vi "Read Config.vi"(8 "error in (no error)":errorcluster, 11 "MQTTclient in":refnum<class "MQTTclient.lvclass">) -> (0 "error out":errorcluster, 2 "Config":T1, 3 "MQTTclient out":refnum<class "MQTTclient.lvclass">)   [LabVIEW 2015, in "MQTTclient.lvclass"]
uses:
  MQTTclient.lvclass
  config.ctl
  MQTTclient.lvclass/MQTTclient.ctl
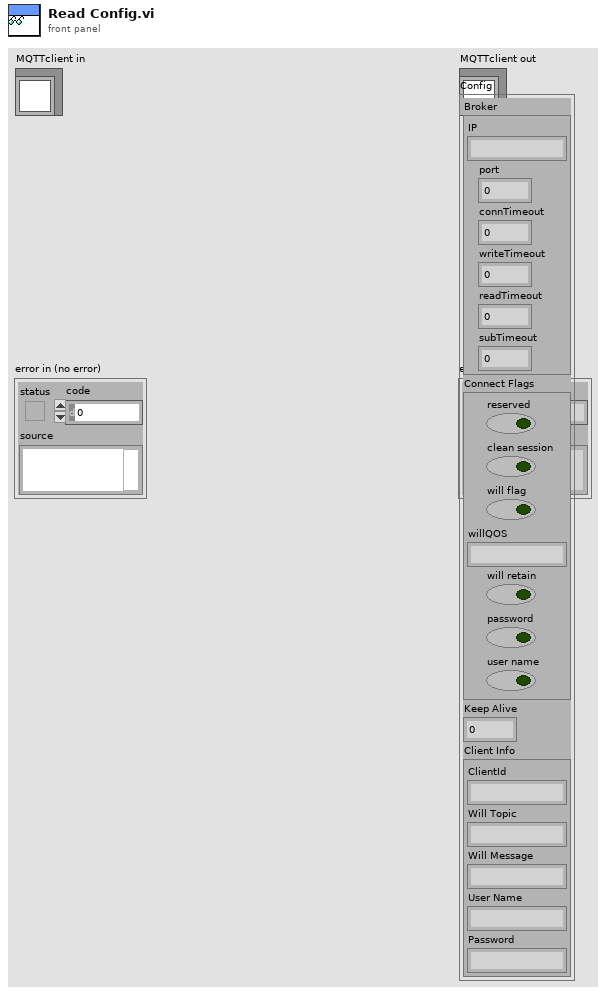
[diagram p1: front panel]
types:
  T1 = typedef "MQTTclient.lvclass/config.ctl" = cluster{"Broker":cluster{"IP":string, "port":u16, "connTimeout":i32, "writeTimeout":i32, "readTimeout":i32, "subTimeout":i32}, "Connect Flags":cluster{"reserved":bool, "clean session":bool, "will flag":bool, "willQOS":string, "will retain":bool, "password":bool, "user name":bool}, "Keep Alive":u16, "Client Info":cluster{"ClientId":string, "Will Topic":string, "Will Message":string, "User Name":string, "Password":string}}
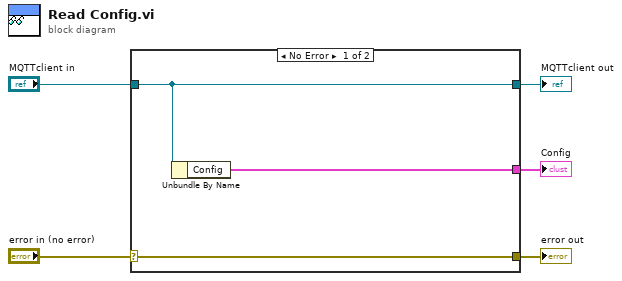
[diagram p0: block diagram]
diagram:
  n1 = case shown="No Error" "error in (no error)" {
    selector: "error in (no error)" -> [w8 w9]
    tunnel: [w8 w9] -> w4
    tunnel: [w7 w10] -> w2
    tunnel: "MQTTclient in" -> [w7 w10]
    tunnel: [w6 _] -> w1
    frame No Error {
      n2 = Unbundle By Name(w7) -> ("Config"=w6:T1)
    }
    frame Error {
    }
  }
  "error out" <- w4
  "MQTTclient out" <- w2
  "Config" <- w1
